vi "destroy.vi"(8 "error in (no error)":errorcluster) -> (0 "error out":errorcluster)   [LabVIEW 2010, in "BalloonNotifier.lvclass"]
uses:
  BalloonNotifier.lvclass
  System.Windows.Forms
panel:
  in  "milliseconds to wait":u32=3000
  in  "notify icon reference":refnum<k24>
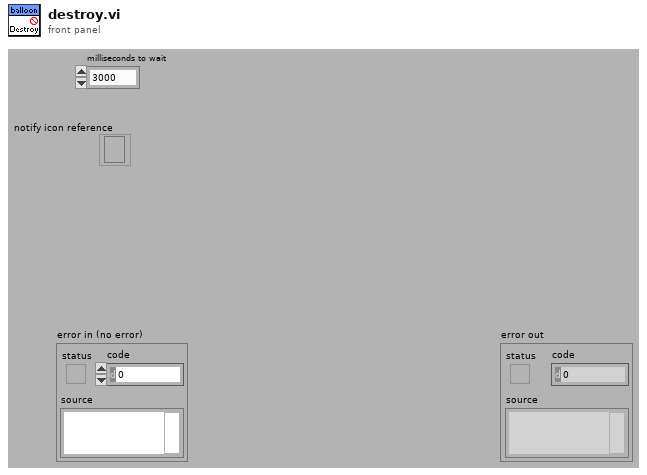
[diagram p1: front panel]
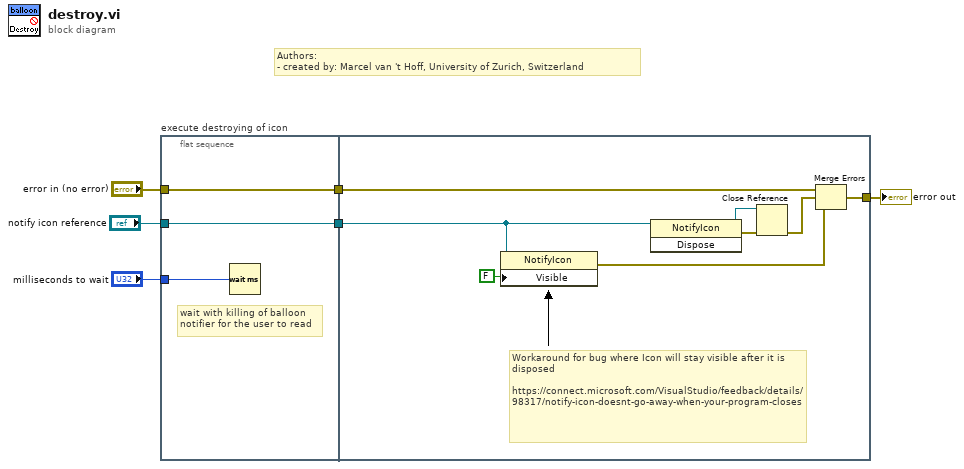
[diagram p0: block diagram]
diagram:
  # "Authors: \n- created by: Marcel van 't Hoff, University of Zurich, Switzerland"
  n1 = flat-sequence "execute destroying of icon" {
    tunnel: "error in (no error)" -> [w9]
    tunnel: [w9] -> w5
    tunnel: "milliseconds to wait" -> [w8]
    tunnel: [w7] -> w2
    tunnel: "notify icon reference" -> [w7]
    tunnel: [w14] -> w6
    tunnel: w5 -> [w11]
    tunnel: w2 -> [w10]
    frame #0 {
      # "wait with killing of balloon\nnotifier for the user to read"
      n2 = Wait (ms)(milliseconds to wait=w8) -> ()  [unwired: 1 out]
    }
    frame #1 {
      # "Workaround for bug where Icon will stay visible after it is disposed\n\nhttps://connect.microsoft.com/VisualStudio/feedback/details/98317/notify-icon-doesnt-go-away-when-your-program-closes"
      n3 = property class="NotifyIcon"(reference=w10, "Visible"=FALSE) -> (error out=w17:errorcluster)  [unwired: 1 in, 1 out]
      n4 = invoke class="NotifyIcon" method="Dispose"(reference=w10) -> (reference out=w16:refnum<k24>, error out=w15:errorcluster)  [unwired: 2 in, 1 out]
      n5 = Close Reference(reference=w16, error in (no error)=w15) -> (error out=w12:errorcluster)
      n6 = Merge Errors(w11, w12, w17) -> (w14:errorcluster)
    }
  }
  "error out" <- w6
